vi "Untitled 11 (SubVI).vi"(7 "error out 4":errorcluster, 8 "error in (no error)":errorcluster, 10 "new file path (Not A Path if cancelled)":path, 11 "Refnum in":refnum<k21>) -> (0 "error out":errorcluster, 1 "DAQ?":bool, 2 "error out":errorcluster, 3 "Refnum out":refnum<k21>, 4 "Available Elements for Reading":i32, 5 "error out 3":errorcluster, 6 "Number of Disconnections":u32)   [LabVIEW 2017]
uses:
  <resource>/objmgr/ni.dex.rc
  <vilib>/Utility/file.llb/Write Delimited Spreadsheet (DBL).vi
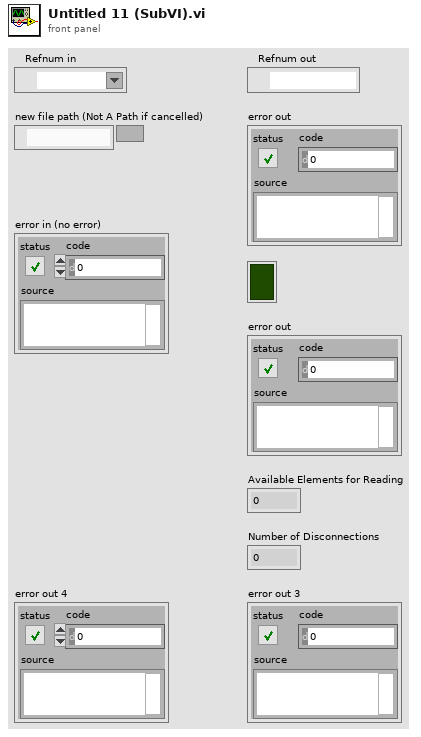
[diagram p1: front panel]
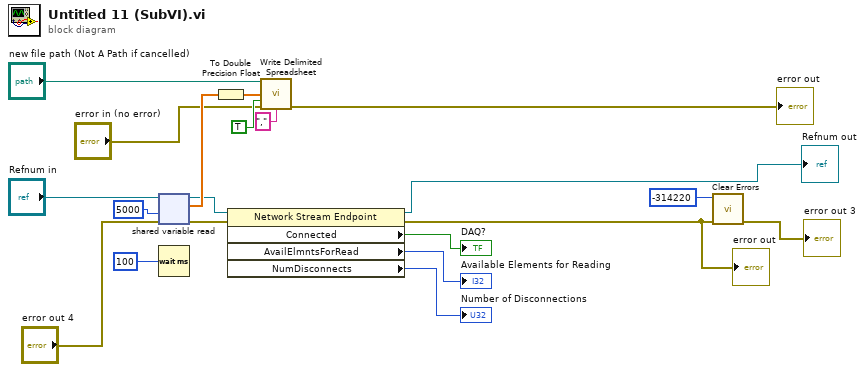
[diagram p0: block diagram]
diagram:
  n1 = shared-variable-read("Refnum in", "error out 4", 5000 ("timeout ms (-1)")) -> (w6:refnum<k21>, w7:errorcluster, w17:sgl[])  [unwired: 1 out]
  n2 = Wait (ms)(milliseconds to wait=u32 100) -> ()  [unwired: 1 out]
  n3 = To Double Precision Float(number=w17) -> (double precision float=w20:dbl[])
  n4 = property class="Network Stream Endpoint"(reference=w6, error in=w7) -> (reference out=→"Refnum out":refnum<k21>, error out=w1:errorcluster, "Connected"=→"DAQ?":bool, "AvailElmntsForRead"=→"Available Elements for Reading":i32, "NumDisconnects"=→"Number of Disconnections":u32)
  "error out" <- w1
  n5 = call-poly <vilib>:"Write Delimited Spreadsheet.vi"("file path (dialog if empty)"="new file path (Not A Path if cancelled)", "1D data"=w20, "append to file? (new file:F)"=TRUE, "error in (no error)"="error in (no error)", "delimiter (\\t)"="," ("delimiter (\\t)")) -> ("error out"=→"error out":errorcluster)  [unwired: 9 in, 1 out]
  n6 = call <vilib>:"Clear Errors.vi"("error in (no error)"=w1, "specific error code to clear (0: all)"=-314220) -> ("error out"=→"error out 3":errorcluster)  [unwired: 4 in, 1 out]
